vi "Resize Block Diagram.vi"(0 "VI in":refnum<vi>, 11 "error in":errorcluster) -> (4 "VI out":refnum<vi>, 15 "error out":errorcluster)   [LabVIEW 2017, in "Align To Connector.lvlib"]
uses:
  Align To Connector.lvlib
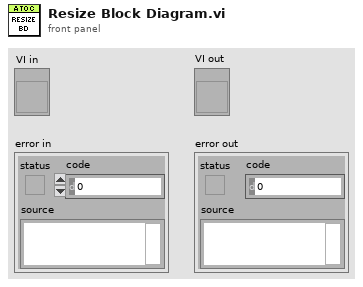
[diagram p1: front panel]
types:
  T1 = cluster{"left":i16, "top":i16, "right":i16, "bottom":i16}
  T2 = typedef "LVRectTypeDef.ctl" = cluster{"Left":i16, "Top":i16, "Right":i16, "Bottom":i16}
  T3 = typedef "LVPointTypeDef.ctl" = cluster{"Horizontal":i16, "Vertical":i16}
  T4 = typedef "LVBoundsTypeDef.ctl" = cluster{"Width":u32, "Height":u32}
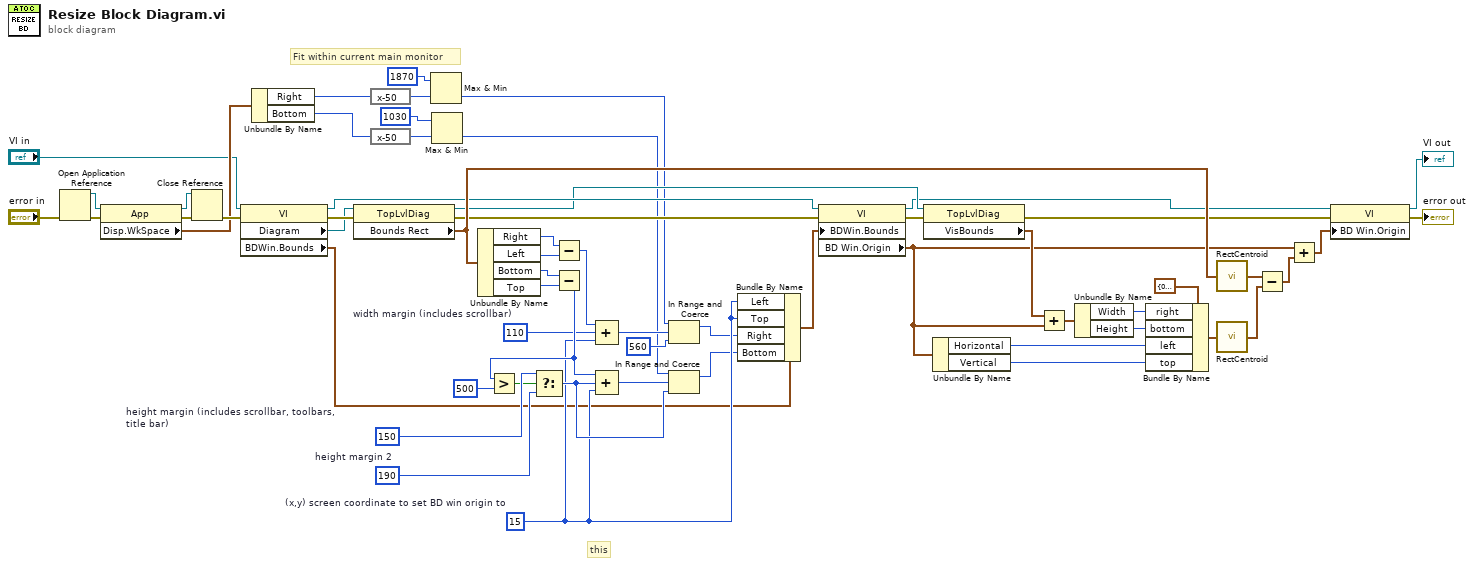
[diagram p0: block diagram]
diagram:
  w56 = i16 190  # height margin 2
  w52 = i16 15  # (x,y) screen coordinate to set BD win origin to
  w55 = i16 150  # height margin (includes scrollbar, toolbars, title bar)
  w47 = i16 110  # width margin (includes scrollbar)
  # "this"
  # "Fit within current main monitor"
  n1 = Open Application Reference() -> (0:w12:errorcluster, 3:w14:refnum<vi>)  [unwired: 4 in]
  n2 = property class="App"(reference=w14, error in=w12) -> (reference out=w2:refnum<vi>, error out=w13:errorcluster, "Disp.WkSpace"=w3:T2)
  n3 = Close Reference(reference=w2, error in (no error)=w13) -> ()  [unwired: 1 out]
  n4 = property on="Property Node" class="VI"(reference="VI in", error in="error in") -> (reference out=w50:refnum<vi>, error out=w51:errorcluster, "Diagram"=w29:refnum<vi>, "BDWin.Bounds"=w16:T2)
  n5 = Unbundle By Name(w3) -> ("Right"=w11:i16, "Bottom"=w10:i16)
  n6 = property on="Property Node" class="TopLvlDiag"(reference=w29, error in=w51) -> (reference out=w45:refnum<vi>, error out=w49:errorcluster, "Bounds Rect"=w53:T2)
  n7 = expression code="x-50"(w11) -> (w9:i16)
  n8 = expression code="x-50"(w10) -> (w7:i16)
  n9 = Max & Min(x=i16 1870 ("upper limit"), y=w9) -> (min(x,y)=w5:i16)  [unwired: 1 out]
  n10 = Max & Min(x=i16 1030 ("upper limit"), y=w7) -> (min(x,y)=w4:i16)  [unwired: 1 out]
  n11 = Unbundle By Name(w53) -> ("Right"=w26:i16, "Left"=w25:i16, "Bottom"=w28:i16, "Top"=w27:i16)
  n12 = Subtract(x=w26, y=w25) -> (x-y=w24:i16)
  n13 = Subtract(x=w28, y=w27) -> (x-y=w58:i16)
  n14 = Greater?(x=w58, y=i16 500) -> (0:w54:bool)
  n15 = Select(t=w55, s=w54, f=w56) -> (s? t:f=w57:i16)
  n16 = Compound Arithmetic op=ADD(w24, w47, w52) -> (w22:i16)
  n17 = Compound Arithmetic op=ADD(w58, w57, w52) -> (w23:i16)
  n18 = In Range and Coerce(upper limit=w5, x=w22, lower limit=i16 560) -> (coerced(x)=w21:i16)  [unwired: 1 out]
  n19 = In Range and Coerce(upper limit=w4, x=w23, lower limit=w57) -> (coerced(x)=w20:i16)  [unwired: 1 out]
  n20 = Bundle By Name(cluster=w16, "Left"=w52, "Top"=w52, "Right"=w21, "Bottom"=w20) -> (w48:T2)
  n21 = property on="Property Node" class="VI"(reference=w50, error in=w49, "BDWin.Bounds"=w48) -> (reference out=w33:refnum<vi>, error out=w46:errorcluster, "BD Win.Origin"=w30:T3)
  n22 = property on="Property Node" class="TopLvlDiag"(reference=w45, error in=w46) -> (error out=w34:errorcluster, "VisBounds"=w41:T4)  [unwired: 1 out]
  n23 = Unbundle By Name(w30) -> ("Horizontal"=w43:i16, "Vertical"=w42:i16)
  n24 = Add(x=w41, y=w30) -> (x+y=w39:T4)
  n25 = Unbundle By Name(w39) -> ("Width"=w40:u32, "Height"=w38:u32)
  n26 = Bundle By Name(cluster=T1 {"left"=0, "top"=0, "right"=0, "bottom"=0} ("rect"), "right"=w40, "bottom"=w38, "left"=w43, "top"=w42) -> (w37:T1)
  n27 = call <vilib>:"RectCentroid.vi"("rect"=w53) -> ("point"=w35:cluster{"x":i16, "y":i16})
  n28 = call <vilib>:"RectCentroid.vi"("rect"=w37) -> ("point"=w36:cluster{"x":i16, "y":i16})
  n29 = Subtract(x=w35, y=w36) -> (x-y=w31:cluster{"x":i16, "y":i16})
  n30 = Add(x=w30, y=w31) -> (x+y=w32:T3)
  n31 = property on="Property Node" class="VI"(reference=w33, error in=w34, "BD Win.Origin"=w32) -> (reference out=→"VI out":refnum<vi>, error out=→"error out":errorcluster)
